vi "do connect to pane.vi"(8 "error in (no error)":errorcluster, 10 "connect_to_pane Argument":T2, 11 "Data Cluster in":T1) -> (0 "error out":errorcluster, 3 "Data Cluster out":T1)   [LabVIEW 2025, in "Scripting Server.lvlib"]
uses:
  Scripting Server.lvlib
  connect_to_pane (Reply Payload)--cluster.ctl
  connect_to_pane Argument--cluster.ctl
  Module Data--cluster.ctl
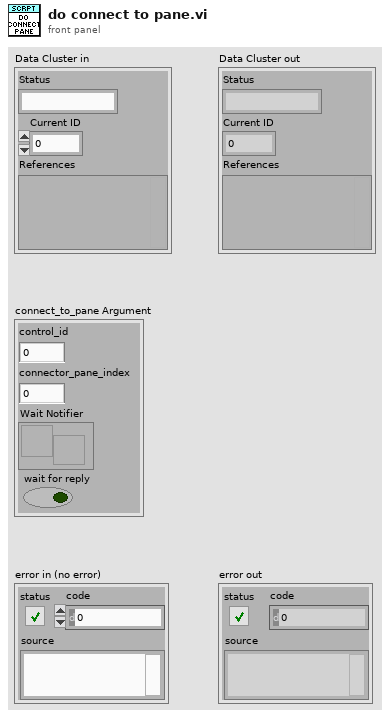
[diagram p1: front panel]
types:
  T1 = typedef "Scripting Server.lvlib/Module Data--cluster.ctl" = cluster{"Status":string, "Current ID":i32, "References":variant}
  T2 = typedef "Scripting Server.lvlib/connect_to_pane Argument--cluster.ctl" = cluster{"control_id":i32, "connector_pane_index":i32, "Wait Notifier":refnum<notifier>, "wait for reply":bool}
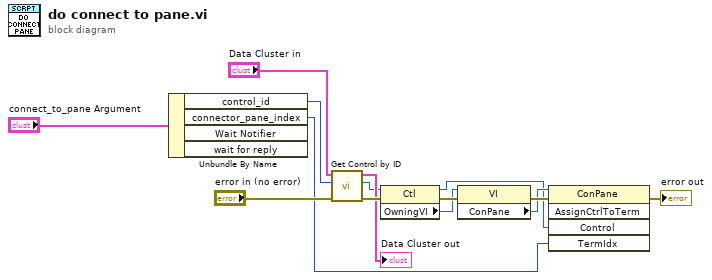
[diagram p0: block diagram]
diagram:
  n1 = Unbundle By Name("connect_to_pane Argument") -> ("control_id"=w9:i32, "connector_pane_index"=w2:i32)  [unwired: 2 out]
  n2 = call "Get Control by ID.vi"("error in (no error)"="error in (no error)", "ID"=w9, "Data Cluster in"="Data Cluster in") -> ("error out"=w12:errorcluster, "specific class reference"=w7:refnum<vi>, "Data Cluster out"=→"Data Cluster out":T1)  [unwired: 6 in]
  n3 = property class="Ctl"(reference=w7, error in=w12) -> (reference out=w1:refnum<vi>, error out=w8:errorcluster, "OwningVI"=w5:refnum<vi>)
  n4 = property class="VI"(reference=w5, error in=w8) -> (error out=w6:errorcluster, "ConPane"=w3:refnum<vi>)  [unwired: 1 out]
  n5 = invoke class="ConPane" method="AssignCtrlToTerm"(reference=w3, error in=w6, "Control"=w1, "TermIdx"=w2) -> (error out=→"error out":errorcluster)  [unwired: 1 in, 4 out]
